vi "CRYTitle bar update.vi"(10 "Step name":string, 11 "Editor VI path":path) -> ()   [LabVIEW 2013]
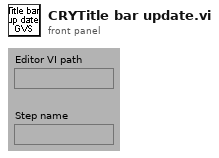
[diagram p1: front panel]
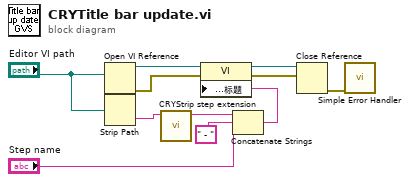
[diagram p0: block diagram]
diagram:
  n1 = Open VI Reference(vi path="Editor VI path") -> (vi reference=w3:refnum<vi>, error out=w4:errorcluster)  [unwired: 1 in, 4 out]
  n2 = Strip Path(path="Editor VI path") -> (name=w8:string)  [unwired: 1 out]
  n3 = call "CRYStrip step extension.vi"("Step name w/ extension"=w8) -> ("Step name (base)"=w9:string)  [unwired: 7 in, 3 out]
  n4 = Concatenate Strings(w9, " - ", "Step name") -> (w11:string)
  n5 = property class="VI"(reference=w3, error in=w4, "前面板窗口:标题"=w11) -> (reference out=w5:refnum<vi>, error out=w6:errorcluster)
  n6 = Close Reference(reference=w5, error in (no error)=w6) -> (error out=w7:errorcluster)
  n7 = call <vilib>:"Simple Error Handler.vi"("error in (no error)"=w7) -> ()  [unwired: 1 in, 8 out]
